vi "Init.vi"(8 "error in (no error)":errorcluster, 11 "PM_Group in":refnum<class "PM_Group.lvclass">) -> (0 "error out":errorcluster, 3 "PM_Group out":refnum<class "PM_Group.lvclass">)   [LabVIEW 2019, in "PM_Group.lvclass"]
uses:
  PM_Group.lvclass
  C:/Users/H4001/Documents/GitHub/H4000/src/Device_class/Device.lvclass
  C:/Users/H4001/Documents/GitHub/H4000/src/Proccess_class/Proccess.lvclass
  Engine_1DO_2DI_class/Config.ctl
  PM_Group.lvclass/PM_Group.ctl
  FPGA/TypeDef/DO index.ctl
  FPGA/TypeDef/DI index.ctl
  Proccess_class/Proccess.lvclass/Proccess.ctl
  Device_class/Device.lvclass/Device.ctl
  Engine_1DO_2DI_class/Engine_1DO_2DI.lvclass/Engine_1DO_2DI.ctl
  Sig_DA_class/Sig_DA.lvclass/Sig_DA.ctl
  SV_Puplisher_class/SV_Publisher.lvclass
  MessageInterface_class/MessageInterface.lvclass
  Sig_DA_class/Write bool_setting.vi
  Engine_1DO_2DI_class/Engine_1DO_2DI.lvclass
  Proccess_class/Proccess.lvclass
  Device_class/Device.lvclass
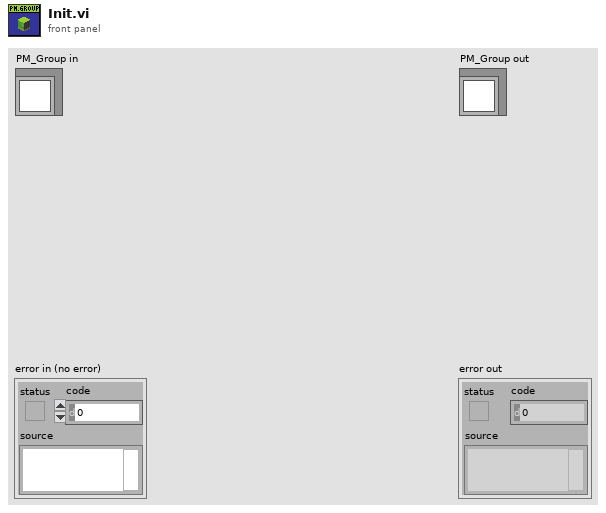
[diagram p1: front panel]
types:
  T1 = typedef "Engine_1DO_2DI.lvclass/Config.ctl" = cluster{"ON_TIMEOUT_MS":dbl, "OFF_TIMEOUT_MS":dbl}
  T2 = typedef "DI index.ctl" = u8
  T3 = typedef "DO index.ctl" = u8
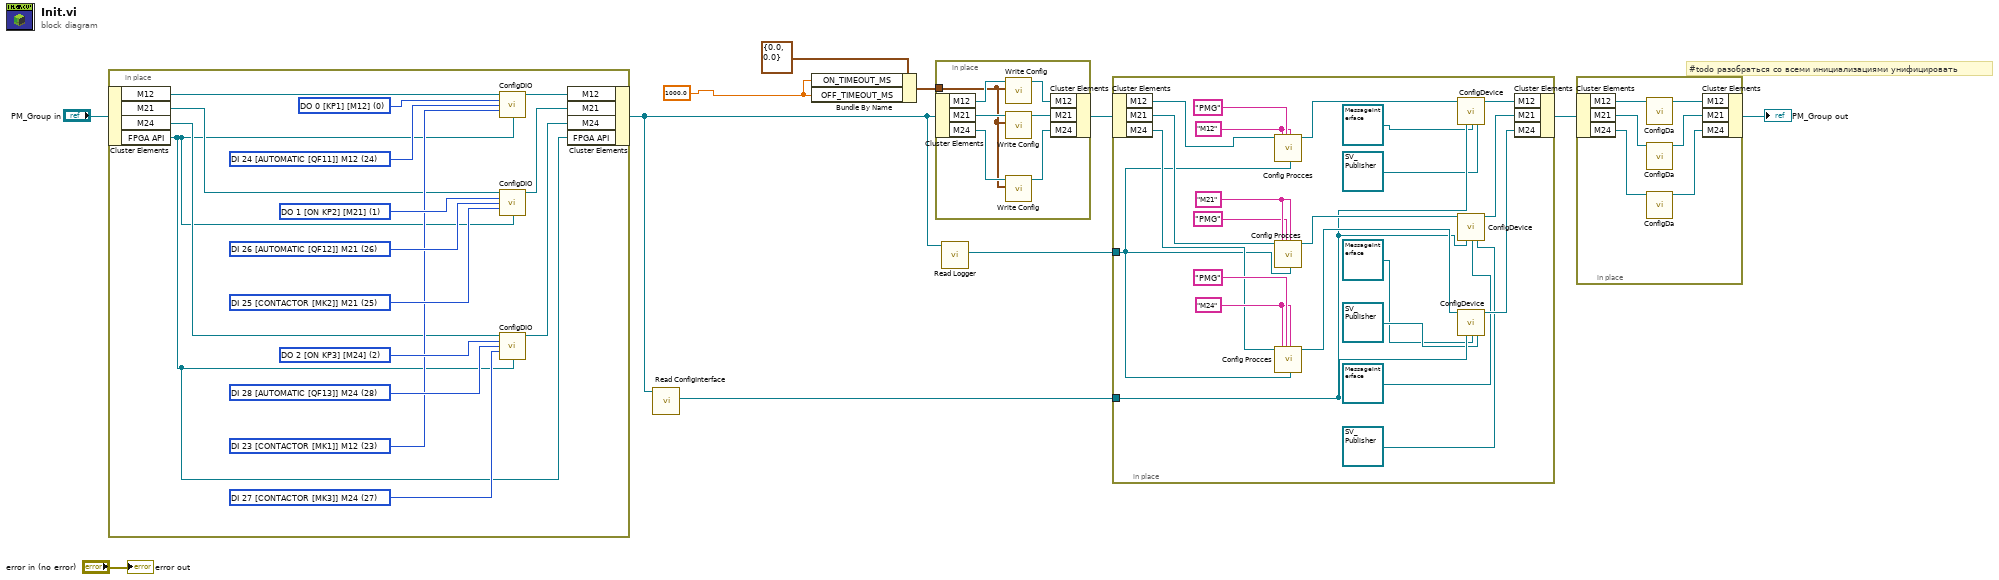
[diagram p0: block diagram]
diagram:
  w1 = 1000.0 ("ON_TIMEOUT_MS")
  # "#todo разобраться со всеми инициализациями унифицировать"
  n1 = in-place {
    w25 = T2 27 items=["DI 0 [QF1]", "DI 1 [QF2]", "DI 2 [QF3]", "DI 3 [QF4]", "DI 4 [QF5]", "DI 5 [QF6]", "DI 6 [QF7]", "DI 7 [QF8]", "DI 8 [QF9]", "DI 9 [PHASE CONTROL RELAY CONTACTOR [KV1]]", "DI 10 [G1]", "DI 11 [G2]", "DI 12 [RESET BTN [SB1]]", "DI 13 [START BTN [SB2]]", "DI 14 [STOP BTN [SB3]]", "DI 15 [ES BTN [SB4]]", "DI 16 [MANUAL/AUTO MODE SA1]", "DI 17 [[S1]]", "DI 18 [[S2]]", "DI 19 [[S3]]", "DI 20 [[S4]]", "DI 21 [44.1 OPEN]", "DI 22 [44.1 CLOSE]", "DI 23 [CONTACTOR [MK1]] M12", "DI 24 [AUTOMATIC [QF11]] M12", "DI 25 [CONTACTOR [MK2]] M21", "DI 26 [AUTOMATIC [QF12]] M21", "DI 27 [CONTACTOR [MK3]] M24", "DI 28 [AUTOMATIC [QF13]] M24", "DI 29 [44.2 OPEN]", "DI 30 [44.2 CLOSE]"] ("DI index")
    w26 = T2 28 items=["DI 0 [QF1]", "DI 1 [QF2]", "DI 2 [QF3]", "DI 3 [QF4]", "DI 4 [QF5]", "DI 5 [QF6]", "DI 6 [QF7]", "DI 7 [QF8]", "DI 8 [QF9]", "DI 9 [PHASE CONTROL RELAY CONTACTOR [KV1]]", "DI 10 [G1]", "DI 11 [G2]", "DI 12 [RESET BTN [SB1]]", "DI 13 [START BTN [SB2]]", "DI 14 [STOP BTN [SB3]]", "DI 15 [ES BTN [SB4]]", "DI 16 [MANUAL/AUTO MODE SA1]", "DI 17 [[S1]]", "DI 18 [[S2]]", "DI 19 [[S3]]", "DI 20 [[S4]]", "DI 21 [44.1 OPEN]", "DI 22 [44.1 CLOSE]", "DI 23 [CONTACTOR [MK1]] M12", "DI 24 [AUTOMATIC [QF11]] M12", "DI 25 [CONTACTOR [MK2]] M21", "DI 26 [AUTOMATIC [QF12]] M21", "DI 27 [CONTACTOR [MK3]] M24", "DI 28 [AUTOMATIC [QF13]] M24", "DI 29 [44.2 OPEN]", "DI 30 [44.2 CLOSE]"] ("DI index")
    w22 = T2 25 items=["DI 0 [QF1]", "DI 1 [QF2]", "DI 2 [QF3]", "DI 3 [QF4]", "DI 4 [QF5]", "DI 5 [QF6]", "DI 6 [QF7]", "DI 7 [QF8]", "DI 8 [QF9]", "DI 9 [PHASE CONTROL RELAY CONTACTOR [KV1]]", "DI 10 [G1]", "DI 11 [G2]", "DI 12 [RESET BTN [SB1]]", "DI 13 [START BTN [SB2]]", "DI 14 [STOP BTN [SB3]]", "DI 15 [ES BTN [SB4]]", "DI 16 [MANUAL/AUTO MODE SA1]", "DI 17 [[S1]]", "DI 18 [[S2]]", "DI 19 [[S3]]", "DI 20 [[S4]]", "DI 21 [44.1 OPEN]", "DI 22 [44.1 CLOSE]", "DI 23 [CONTACTOR [MK1]] M12", "DI 24 [AUTOMATIC [QF11]] M12", "DI 25 [CONTACTOR [MK2]] M21", "DI 26 [AUTOMATIC [QF12]] M21", "DI 27 [CONTACTOR [MK3]] M24", "DI 28 [AUTOMATIC [QF13]] M24", "DI 29 [44.2 OPEN]", "DI 30 [44.2 CLOSE]"] ("DI index")
    w23 = T2 26 items=["DI 0 [QF1]", "DI 1 [QF2]", "DI 2 [QF3]", "DI 3 [QF4]", "DI 4 [QF5]", "DI 5 [QF6]", "DI 6 [QF7]", "DI 7 [QF8]", "DI 8 [QF9]", "DI 9 [PHASE CONTROL RELAY CONTACTOR [KV1]]", "DI 10 [G1]", "DI 11 [G2]", "DI 12 [RESET BTN [SB1]]", "DI 13 [START BTN [SB2]]", "DI 14 [STOP BTN [SB3]]", "DI 15 [ES BTN [SB4]]", "DI 16 [MANUAL/AUTO MODE SA1]", "DI 17 [[S1]]", "DI 18 [[S2]]", "DI 19 [[S3]]", "DI 20 [[S4]]", "DI 21 [44.1 OPEN]", "DI 22 [44.1 CLOSE]", "DI 23 [CONTACTOR [MK1]] M12", "DI 24 [AUTOMATIC [QF11]] M12", "DI 25 [CONTACTOR [MK2]] M21", "DI 26 [AUTOMATIC [QF12]] M21", "DI 27 [CONTACTOR [MK3]] M24", "DI 28 [AUTOMATIC [QF13]] M24", "DI 29 [44.2 OPEN]", "DI 30 [44.2 CLOSE]"] ("DI index")
    w19 = T2 23 items=["DI 0 [QF1]", "DI 1 [QF2]", "DI 2 [QF3]", "DI 3 [QF4]", "DI 4 [QF5]", "DI 5 [QF6]", "DI 6 [QF7]", "DI 7 [QF8]", "DI 8 [QF9]", "DI 9 [PHASE CONTROL RELAY CONTACTOR [KV1]]", "DI 10 [G1]", "DI 11 [G2]", "DI 12 [RESET BTN [SB1]]", "DI 13 [START BTN [SB2]]", "DI 14 [STOP BTN [SB3]]", "DI 15 [ES BTN [SB4]]", "DI 16 [MANUAL/AUTO MODE SA1]", "DI 17 [[S1]]", "DI 18 [[S2]]", "DI 19 [[S3]]", "DI 20 [[S4]]", "DI 21 [44.1 OPEN]", "DI 22 [44.1 CLOSE]", "DI 23 [CONTACTOR [MK1]] M12", "DI 24 [AUTOMATIC [QF11]] M12", "DI 25 [CONTACTOR [MK2]] M21", "DI 26 [AUTOMATIC [QF12]] M21", "DI 27 [CONTACTOR [MK3]] M24", "DI 28 [AUTOMATIC [QF13]] M24", "DI 29 [44.2 OPEN]", "DI 30 [44.2 CLOSE]"] ("DI index")
    w20 = T2 24 items=["DI 0 [QF1]", "DI 1 [QF2]", "DI 2 [QF3]", "DI 3 [QF4]", "DI 4 [QF5]", "DI 5 [QF6]", "DI 6 [QF7]", "DI 7 [QF8]", "DI 8 [QF9]", "DI 9 [PHASE CONTROL RELAY CONTACTOR [KV1]]", "DI 10 [G1]", "DI 11 [G2]", "DI 12 [RESET BTN [SB1]]", "DI 13 [START BTN [SB2]]", "DI 14 [STOP BTN [SB3]]", "DI 15 [ES BTN [SB4]]", "DI 16 [MANUAL/AUTO MODE SA1]", "DI 17 [[S1]]", "DI 18 [[S2]]", "DI 19 [[S3]]", "DI 20 [[S4]]", "DI 21 [44.1 OPEN]", "DI 22 [44.1 CLOSE]", "DI 23 [CONTACTOR [MK1]] M12", "DI 24 [AUTOMATIC [QF11]] M12", "DI 25 [CONTACTOR [MK2]] M21", "DI 26 [AUTOMATIC [QF12]] M21", "DI 27 [CONTACTOR [MK3]] M24", "DI 28 [AUTOMATIC [QF13]] M24", "DI 29 [44.2 OPEN]", "DI 30 [44.2 CLOSE]"] ("DI index")
    w27 = T3 2 items=["DO 0 [KP1] [M12]", "DO 1 [ON KP2] [M21]", "DO 2 [ON KP3] [M24]", "DO 3 [WATER Y18.1 [DO3]]", "DO 4 [WATER Y18.2 [DO4]]", "DO 5 [KP6 Y29.1 33.7]", "DO 6 [KP7 Y29.2 33.8]", "DO 7 [KP8 Y29.3 33.9]", "DO 8 [KP9 Y29.4  33.12]", "DO 9 [KP10 Y29.5 33.1]", "DO 10 [KP11 Y29.6 33.2]", "DO 11 [KP12 Y29.7  33.13]", "DO 12 [KP13 Y29.8  33.11]", "DO 13 [KP14 Y29.9 33.10]", "DO 14 [KP15 Y29.10  33.6]", "DO 15 [KP16 Y29.11  33.5]", "DO 16 [KP17 Y29.12  33.4]", "DO 17 [KP18 Y29.13 33.3]", "DO 18 [AIR KP19]", "DO 19 [STEP DRIVE EN KP20]", "DO 20 [KP21 Y44.1 OPEN]", "DO 21 [ KP22 Y44.1 CLOSE]", "DO 22 [ KP23 Y44.2 OPEN]", "DO 23", "DO 24 [STEP DRIVE 1]", "DO 25 [STEP DRIVE 2]"] ("DO index")
    w24 = T3 1 items=["DO 0 [KP1] [M12]", "DO 1 [ON KP2] [M21]", "DO 2 [ON KP3] [M24]", "DO 3 [WATER Y18.1 [DO3]]", "DO 4 [WATER Y18.2 [DO4]]", "DO 5 [KP6 Y29.1 33.7]", "DO 6 [KP7 Y29.2 33.8]", "DO 7 [KP8 Y29.3 33.9]", "DO 8 [KP9 Y29.4  33.12]", "DO 9 [KP10 Y29.5 33.1]", "DO 10 [KP11 Y29.6 33.2]", "DO 11 [KP12 Y29.7  33.13]", "DO 12 [KP13 Y29.8  33.11]", "DO 13 [KP14 Y29.9 33.10]", "DO 14 [KP15 Y29.10  33.6]", "DO 15 [KP16 Y29.11  33.5]", "DO 16 [KP17 Y29.12  33.4]", "DO 17 [KP18 Y29.13 33.3]", "DO 18 [AIR KP19]", "DO 19 [STEP DRIVE EN KP20]", "DO 20 [KP21 Y44.1 OPEN]", "DO 21 [ KP22 Y44.1 CLOSE]", "DO 22 [ KP23 Y44.2 OPEN]", "DO 23", "DO 24 [STEP DRIVE 1]", "DO 25 [STEP DRIVE 2]"] ("DO index")
    w21 = T3 0 items=["DO 0 [KP1] [M12]", "DO 1 [ON KP2] [M21]", "DO 2 [ON KP3] [M24]", "DO 3 [WATER Y18.1 [DO3]]", "DO 4 [WATER Y18.2 [DO4]]", "DO 5 [KP6 Y29.1 33.7]", "DO 6 [KP7 Y29.2 33.8]", "DO 7 [KP8 Y29.3 33.9]", "DO 8 [KP9 Y29.4  33.12]", "DO 9 [KP10 Y29.5 33.1]", "DO 10 [KP11 Y29.6 33.2]", "DO 11 [KP12 Y29.7  33.13]", "DO 12 [KP13 Y29.8  33.11]", "DO 13 [KP14 Y29.9 33.10]", "DO 14 [KP15 Y29.10  33.6]", "DO 15 [KP16 Y29.11  33.5]", "DO 16 [KP17 Y29.12  33.4]", "DO 17 [KP18 Y29.13 33.3]", "DO 18 [AIR KP19]", "DO 19 [STEP DRIVE EN KP20]", "DO 20 [KP21 Y44.1 OPEN]", "DO 21 [ KP22 Y44.1 CLOSE]", "DO 22 [ KP23 Y44.2 OPEN]", "DO 23", "DO 24 [STEP DRIVE 1]", "DO 25 [STEP DRIVE 2]"] ("DO index")
    n2 = in-place-cluster #1("PM_Group in") -> ("M12"=w15:refnum<class "Engine_1DO_2DI.lvclass">, "M21"=w14:refnum<class "Engine_1DO_2DI.lvclass">, "M24"=w13:refnum<class "Engine_1DO_2DI.lvclass">, "FPGA API"=w12:refnum<class "FPGA API.lvclass">)
    n3 = call "ConfigDIO.vi"("Pump_1AI_1DO_2DI in"=w15, "DO"=w21, "DI A"=w20, "DI C"=w19, "FPGA API"=w12) -> ("Pump_1AI_1DO_2DI out"=w18:refnum<class "Engine_1DO_2DI.lvclass">)  [unwired: 10 in]
    n4 = call "ConfigDIO.vi"("Pump_1AI_1DO_2DI in"=w14, "DO"=w24, "DI A"=w23, "DI C"=w22, "FPGA API"=w12) -> ("Pump_1AI_1DO_2DI out"=w17:refnum<class "Engine_1DO_2DI.lvclass">)  [unwired: 10 in]
    n5 = call "ConfigDIO.vi"("Pump_1AI_1DO_2DI in"=w13, "DO"=w27, "DI A"=w26, "DI C"=w25, "FPGA API"=w12) -> ("Pump_1AI_1DO_2DI out"=w16:refnum<class "Engine_1DO_2DI.lvclass">)  [unwired: 10 in]
    n6 = in-place-cluster #1("M12"=w18, "M21"=w17, "M24"=w16, "FPGA API"=w12) -> (w6:refnum<class "PM_Group.lvclass">)
  }
  n7 = call "Read ConfigInterface.vi"("Device in"=w6) -> ("ConfigInterface"=w4:refnum<class "ConfigInterface.lvclass">)  [unwired: 10 in]
  n8 = Bundle By Name(cluster=T1 {"ON_TIMEOUT_MS"=0.0, "OFF_TIMEOUT_MS"=0.0} ("Config"), "ON_TIMEOUT_MS"=w1, "OFF_TIMEOUT_MS"=w1) -> (w8:T1)
  n9 = in-place {
    in-place-border: w8 -> [w28]
    n10 = in-place-cluster #2(w6) -> ("M12"=w34:refnum<class "Engine_1DO_2DI.lvclass">, "M21"=w32:refnum<class "Engine_1DO_2DI.lvclass">, "M24"=w29:refnum<class "Engine_1DO_2DI.lvclass">)
    n11 = call "Write Config.vi"("Config"=w28, "Pump_1AI_1DO_2DI in"=w34) -> ("Pump_1AI_1DO_2DI out"=w33:refnum<class "Engine_1DO_2DI.lvclass">)  [unwired: 9 in]
    n12 = call "Write Config.vi"("Config"=w28, "Pump_1AI_1DO_2DI in"=w32) -> ("Pump_1AI_1DO_2DI out"=w31:refnum<class "Engine_1DO_2DI.lvclass">)  [unwired: 9 in]
    n13 = call "Write Config.vi"("Config"=w28, "Pump_1AI_1DO_2DI in"=w29) -> ("Pump_1AI_1DO_2DI out"=w30:refnum<class "Engine_1DO_2DI.lvclass">)  [unwired: 9 in]
    n14 = in-place-cluster #2("M12"=w33, "M21"=w31, "M24"=w30) -> (w7:refnum<class "PM_Group.lvclass">)
  }
  n15 = call "Read Logger.vi"("Proccess in"=w6) -> ("Logger"=w5:refnum<class "Logger.lvclass">)  [unwired: 10 in]
  n16 = in-place {
    in-place-border: w5 -> [w42]
    in-place-border: w4 -> [w41]
    w47 = "M24" ("Name")
    w52 = "M21" ("Name")
    w53 = "M12" ("Name")
    n17 = in-place-cluster #3(w7) -> ("M12"=w55:refnum<class "Engine_1DO_2DI.lvclass">, "M21"=w46:refnum<class "Engine_1DO_2DI.lvclass">, "M24"=w44:refnum<class "Engine_1DO_2DI.lvclass">)
    n18 = call "Config Procces.vi"("reference in"=w55, "Name"=w53, "ParentName"="PMG", "Description"=w53, "Logger"=w42) -> ("reference out"=w56:refnum<class "Engine_1DO_2DI.lvclass">)  [unwired: 13 in, 1 out]
    n19 = call "Config Procces.vi"("reference in"=w46, "Name"=w52, "ParentName"="PMG", "Description"=w52, "Logger"=w42) -> ("reference out"=w51:refnum<class "Engine_1DO_2DI.lvclass">)  [unwired: 13 in, 1 out]
    n20 = call "Config Procces.vi"("reference in"=w44, "Name"=w47, "ParentName"="PMG", "Description"=w47, "Logger"=w42) -> ("reference out"=w48:refnum<class "Engine_1DO_2DI.lvclass">)  [unwired: 13 in, 1 out]
    n21 = call "ConfigDevice.vi"("Device in"=w56, "ConfigInterface"=w41, "MessageInterface"=refnum<class "MessageInterface.lvclass"> refnum, "SV_Publisher"=refnum<class "SV_Publisher.lvclass"> refnum) -> ("Device out"=w54:refnum<class "Engine_1DO_2DI.lvclass">)  [unwired: 11 in]
    n22 = call "ConfigDevice.vi"("Device in"=w51, "ConfigInterface"=w41, "MessageInterface"=refnum<class "MessageInterface.lvclass"> refnum, "SV_Publisher"=refnum<class "SV_Publisher.lvclass"> refnum) -> ("Device out"=w45:refnum<class "Engine_1DO_2DI.lvclass">)  [unwired: 11 in]
    n23 = call "ConfigDevice.vi"("Device in"=w48, "ConfigInterface"=w41, "MessageInterface"=refnum<class "MessageInterface.lvclass"> refnum, "SV_Publisher"=refnum<class "SV_Publisher.lvclass"> refnum) -> ("Device out"=w43:refnum<class "Engine_1DO_2DI.lvclass">)  [unwired: 11 in]
    n24 = in-place-cluster #3("M12"=w54, "M21"=w45, "M24"=w43) -> (w3:refnum<class "PM_Group.lvclass">)
  }
  n25 = in-place {
    n26 = in-place-cluster #4(w3) -> ("M12"=w63:refnum<class "Engine_1DO_2DI.lvclass">, "M21"=w61:refnum<class "Engine_1DO_2DI.lvclass">, "M24"=w60:refnum<class "Engine_1DO_2DI.lvclass">)
    n27 = call "ConfigDa.vi"("Pump_1AI_1DO_2DI in"=w63) -> ("Pump_1AI_1DO_2DI out"=w62:refnum<class "Engine_1DO_2DI.lvclass">)  [unwired: 13 in, 1 out]
    n28 = call "ConfigDa.vi"("Pump_1AI_1DO_2DI in"=w61) -> ("Pump_1AI_1DO_2DI out"=w59:refnum<class "Engine_1DO_2DI.lvclass">)  [unwired: 13 in, 1 out]
    n29 = call "ConfigDa.vi"("Pump_1AI_1DO_2DI in"=w60) -> ("Pump_1AI_1DO_2DI out"=w58:refnum<class "Engine_1DO_2DI.lvclass">)  [unwired: 13 in, 1 out]
    n30 = in-place-cluster #4("M12"=w62, "M21"=w59, "M24"=w58) -> (→"PM_Group out":refnum<class "PM_Group.lvclass">)
  }
  "error out" <- "error in (no error)"
